vi "global_variables.vi"() -> ()   [LabVIEW 2023]
panel:
  in  "humidity-value":dbl[](array[numeric])
  in  "perceived-temperature-value":dbl[](array[numeric])
  in  "temperature-value":dbl[](array[numeric])
  in  "date-time":string[](array[string])
  in  "humidity-report":string[](array[string])
  in  "perceived-temperature-report":string[](array[string])
  in  "temperature-report":string[](array[string])
  in  "all-data-report":string[](array[string])
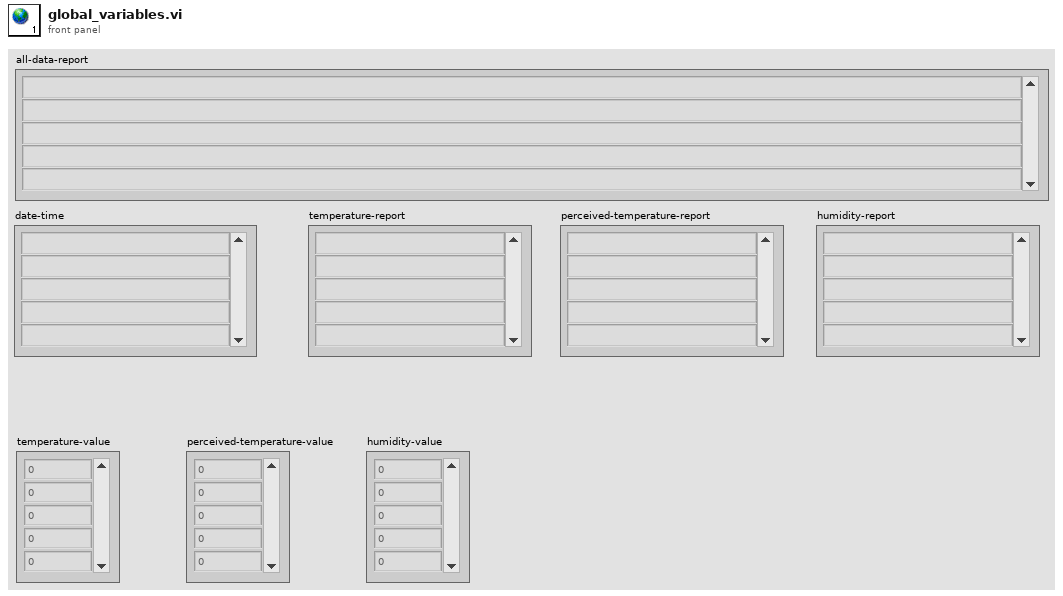
[diagram p1: front panel]
diagram:
